vi "Load.vi"(8 "Error In":errorcluster, 10 "Key":string, 11 "Loader In":refnum<class "String.lvclass">) -> (0 "Error Out":errorcluster, 2 "Template":string, 3 "Loader Out":refnum<class "String.lvclass">)   [LabVIEW 2018, in "Toolkit.lvlib" / "Loaders.lvlib" / "String.lvclass"]
doc: "Gets a template as a string based on the Partial's key value in the root, or master, template."
uses:
  String.lvclass
  String.lvclass/String.ctl
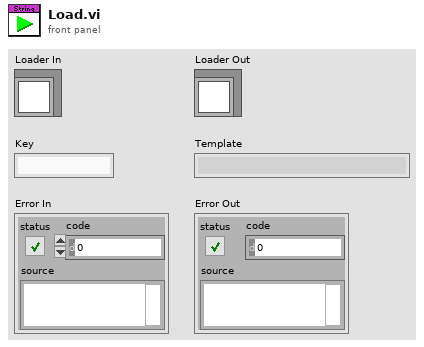
[diagram p1: front panel]
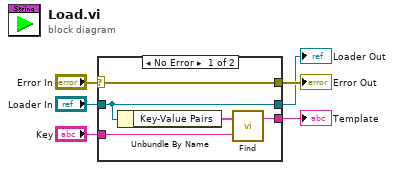
[diagram p0: block diagram]
diagram:
  n1 = case shown="No Error" "Error In" {
    selector: "Error In" -> [w8 w12]
    tunnel: "Loader In" -> [w7 w13]
    tunnel: "Key" -> [w10 _]
    tunnel: [w9 _] -> w3
    tunnel: [w8 w12] -> w2
    tunnel: [w7 w13] -> w1
    frame No Error {
      n2 = Unbundle By Name(w7) -> ("Key-Value Pairs"=w11:cluster{"Key":string, "Value":string}[])
      n3 = call "Find.vi"("Key"=w10, "Key-Value Pairs"=w11) -> ("Value"=w9:string)  [unwired: 1 out]
    }
    frame Error {
    }
  }
  "Loader Out" <- w1
  "Error Out" <- w2
  "Template" <- w3
